vi "LTC20C read sensor 1 v0.3.vi"(2 "Point #":i32, 3 "GPIB\nAddress":refnum<visa-resource-name>) -> (0 "Stop":bool, 1 "Temperature (K)":dbl format="%.2f")   [LabVIEW 2019]
doc: "This VI reads the sample output of the Lakeshore DRC 93C or 82C temperature controller. The output is an array consisting of the single reading. The input is the numeric GPIB address.\nScott Hannahs, F. Bitter National Magnet Lab, 1993"
panel:
  out "Output":dbl[](array[numeric]) format="%.3f"
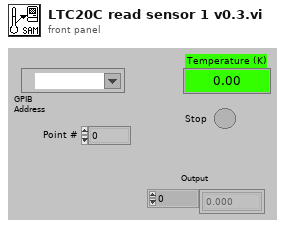
[diagram p1: front panel]
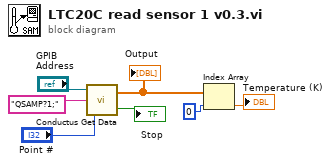
[diagram p0: block diagram]
diagram:
  n1 = call "Conductus Get Data.vi"("Point #"="Point #", "Command String"="QSAMP?1;", "GPIB Address"="GPIB\nAddress") -> ("Stop"=→"Stop":bool, "Measurement"=w2:dbl[])
  "Output" <- w2
  n2 = Index Array(array=w2, index=0) -> (element=→"Temperature (K)":dbl)
